vi "Close.vi"(8 "error in (no error)":errorcluster, 11 "NI PXI Trigger in":refnum<class "NI PXI Trigger.lvclass">) -> (0 "error out":errorcluster, 3 "NI PXI Trigger out":refnum<class "NI PXI Trigger.lvclass">)   [LabVIEW 2020, in "NI DAQmx.lvlib" / "NI PXI Trigger.lvclass"]
uses:
  NI PXI Trigger.lvclass
  NI PXI Trigger.lvclass/NI PXI Trigger.ctl
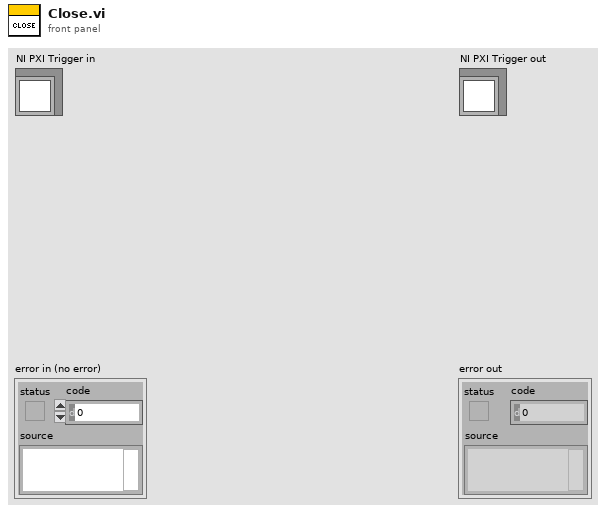
[diagram p1: front panel]
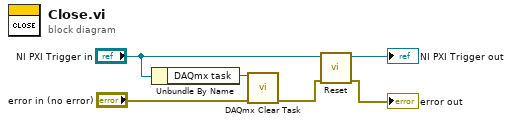
[diagram p0: block diagram]
diagram:
  n1 = Unbundle By Name("NI PXI Trigger in") -> ("DAQmx task"=w4:refnum<k21>)
  n2 = call <vilib>:"DAQmx Clear Task.vi"("task in"=w4, "error in"="error in (no error)") -> ("error out"=w2:errorcluster)  [unwired: 13 in]
  n3 = call-dynamic "Reset.vi"("error in (no error)"=w2, "NI PXI Trigger in"="NI PXI Trigger in") -> ("error out"=→"error out":errorcluster, "NI PXI Trigger out"=→"NI PXI Trigger out":refnum<class "NI PXI Trigger.lvclass">)  [unwired: 8 in]
